vi "Insert Item.vi"(8 "错误输入":errorcluster, 9 "Index":i32, 10 "Item":string[](array[string]), 11 "Mlistbox Ref":refnum<vi>) -> (0 "错误输出":errorcluster, 3 "Mlistbox Ref Dup":refnum<vi>)   [LabVIEW 2012, in "Mlistbox Tools.lvlib"]
uses:
  Mlistbox Tools.lvlib
  ListBox/Custom Type/Read and Write Mode.ctl
  Property/Set and Get ItemNames.vi
  ListBox/Listbox Tool.lvlib
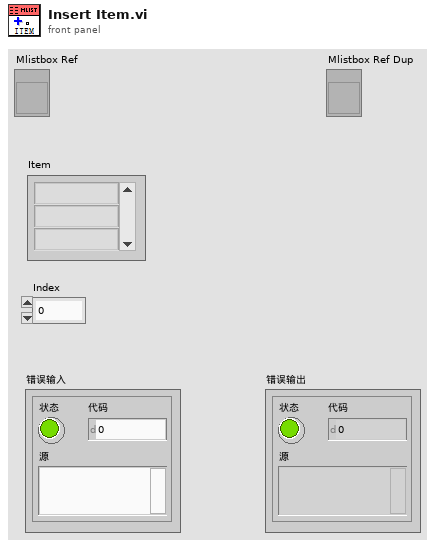
[diagram p1: front panel]
types:
  T1 = typedef "Listbox Tool.lvlib/Read and Write Mode.ctl" = enum16{"Read", "Write"}
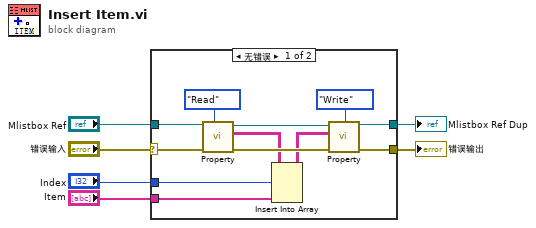
[diagram p0: block diagram]
diagram:
  n1 = case shown="无错误" "错误输入" {
    selector: "错误输入" -> [w15 w20]
    tunnel: [w13 w20] -> w5
    tunnel: "Mlistbox Ref" -> [w18 w19]
    tunnel: "Index" -> [w9 _]
    tunnel: "Item" -> [w8 _]
    tunnel: [w14 w19] -> w2
    frame No Error {
      n2 = call-poly "Property.vi"("Mode"=Read_and_Write_Mode."Read", "错误输入"=w15, "Mlistbox Ref"=w18) -> ("错误输出"=w11:errorcluster, "ItemNames Out"=w10:string[][], "Mlistbox Ref Dup"=w12:refnum<vi>)  [unwired: 6 in]
      n3 = Insert Into Array(array=w10, index (row)=w9, new element=w8) -> (w7:string[][])  [unwired: 1 in]
      n4 = call-poly "Property.vi"("Mode"=Read_and_Write_Mode."Write", "错误输入"=w11, "ItemNames In"=w7, "Mlistbox Ref"=w12) -> ("错误输出"=w13:errorcluster, "Mlistbox Ref Dup"=w14:refnum<vi>)  [unwired: 5 in, 1 out]
    }
    frame Error {
    }
  }
  "Mlistbox Ref Dup" <- w2
  "错误输出" <- w5
